vi "PRTA Log File 2011.vi"(8 "Output File":path) -> (4 "data file":string="Data File:    created on Friday, December 03, 1999  at  4:41:37 PM\n\nWARNING: No tampering with this data please.\n\nTomasz W. Wysokinski   Cryofuel Systems Group © 1997/99.\n\n\n Abs. Time \t Run Time\tHCL-VLT\t HeatPipe \t GM-1 \tunused\t SHLD-1\t GM-2\t HCL-bottom\t M-1\t M-2\t SHLD-2\t Hall-P\t Magnet\r")   [LabVIEW 2010]
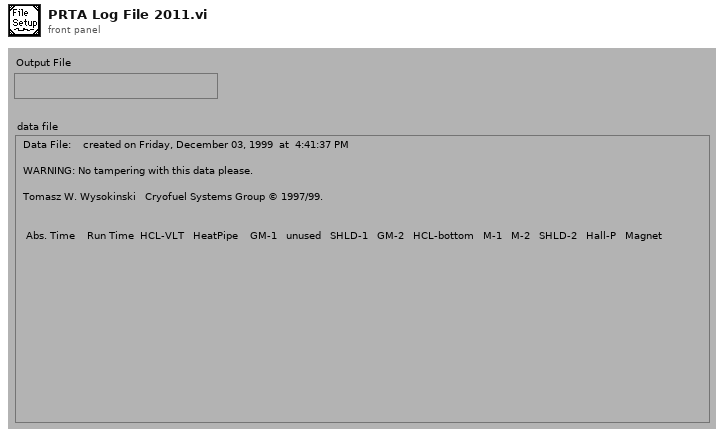
[diagram p1: front panel]
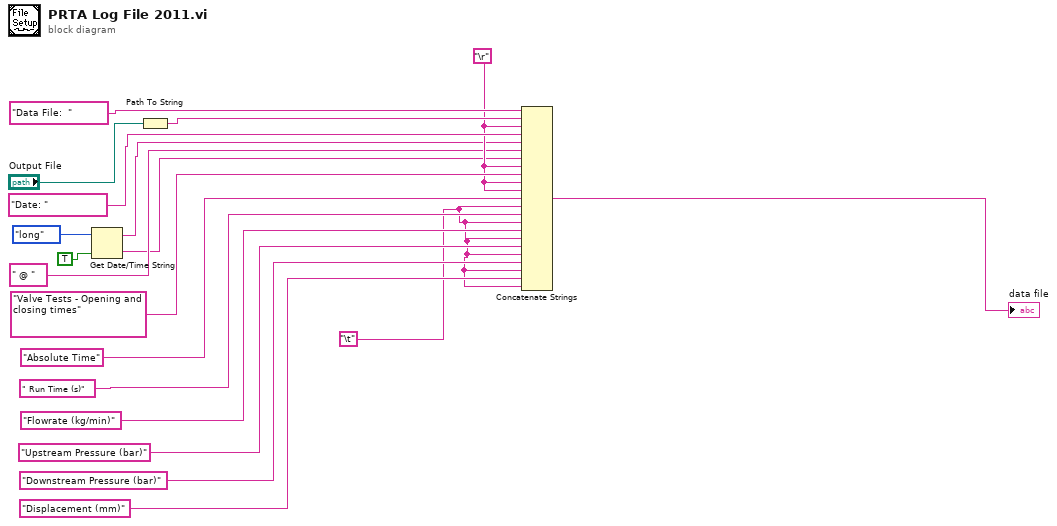
[diagram p0: block diagram]
diagram:
  w1 = "\t" ("time string")
  w6 = "\r"
  n1 = Get Date/Time String(date format (0)=enum16{"short", "long", "abbreviated"}."long", want seconds? (F)=TRUE) -> (date string=w5:string, time string=w3:string)  [unwired: 1 out]
  n2 = Path To String(path="Output File") -> (string=w8:string)
  n3 = Concatenate Strings("Data File:  ", w8, w6, "Date: ", w5, " @ ", w3, w6, "Valve Tests - Opening and closing times", w6, w6, "Absolute Time", w1, " Run Time (s)", w1, "Flowrate (kg/min)", w1, "Upstream Pressure (bar)", w1, "Downstream Pressure (bar)", w1, "Displacement (mm)", w1) -> (→"data file":string)
